vi "Untitled 6 (SubVI).vi"(0 "TestInterface in":refnum<class "TestInterface.lvclass">, 1 "timings":i32[](array[numeric]), 2 "reference 4":refnum<vi>, 3 "parameters":string[][](array[string]), 4 "reference 5":refnum<vi>, 5 "reference 6":refnum<vi>, 6 "reference 7":refnum<vi>, 8 "reference 3":refnum<vi>, 9 "name":string, 10 "response":bool[](array[boolean]), 11 "Command regex":string[](array[string]), 12 "reference 2":refnum<vi>, 13 "Commandlist":string, 14 "reference":refnum<vi>, 16 "wait":u32[](array[numeric])) -> (20 "TestInterface out":refnum<class "TestInterface.lvclass">, 27 "error out":errorcluster)   [LabVIEW 2013, in "DeviceInterface.lvclass"]
uses:
  DeviceInterface.lvclass
  Tests/TestInterface/TestInterface.lvclass
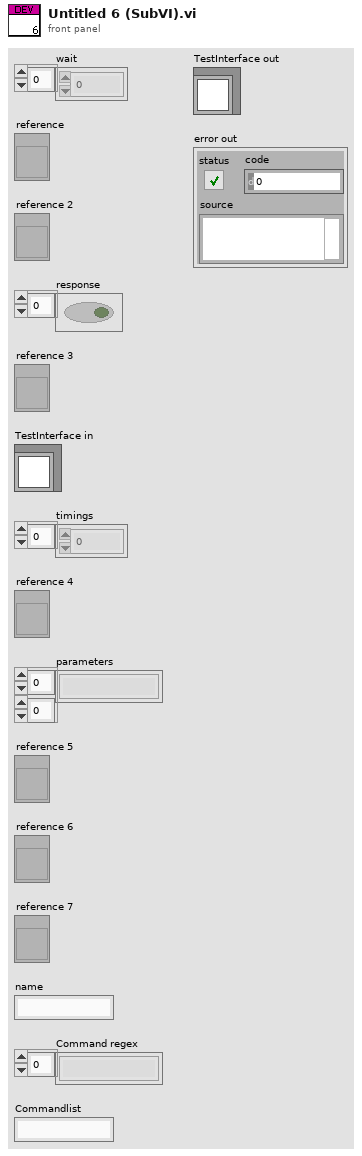
[diagram p1: front panel]
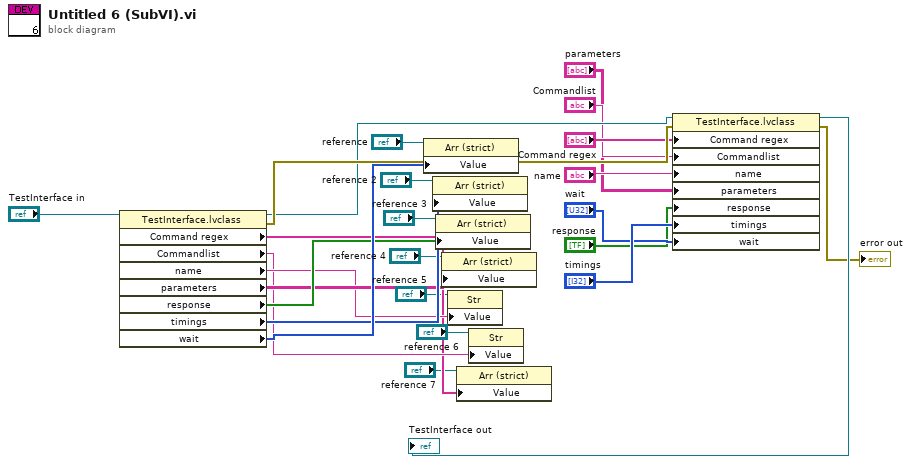
[diagram p0: block diagram]
diagram:
  n1 = property class="TestInterface.lvclass"(reference="TestInterface in") -> (reference out=w23:refnum<class "TestInterface.lvclass">, error out=w24:errorcluster, "Command regex"=w9:string[], "Commandlist"=w10:string, "name"=w11:string, "parameters"=w12:string[][], "response"=w13:bool[], "timings"=w14:i32[], "wait"=w15:u32[])  [unwired: 1 in]
  n2 = property class="Arr (strict)"(reference="reference", "Value"=w15) -> ()  [unwired: 1 in, 2 out]
  n3 = property class="Arr (strict)"(reference="reference 2", "Value"=w14) -> ()  [unwired: 1 in, 2 out]
  n4 = property class="Arr (strict)"(reference="reference 3", "Value"=w13) -> ()  [unwired: 1 in, 2 out]
  n5 = property class="Arr (strict)"(reference="reference 4", "Value"=w12) -> ()  [unwired: 1 in, 2 out]
  n6 = property class="Str"(reference="reference 5", "Value"=w11) -> ()  [unwired: 1 in, 2 out]
  n7 = property class="Arr (strict)"(reference="reference 7", "Value"=w9) -> ()  [unwired: 1 in, 2 out]
  n8 = property class="Str"(reference="reference 6", "Value"=w10) -> ()  [unwired: 1 in, 2 out]
  n9 = property class="TestInterface.lvclass"(reference=w23, error in=w24, "Command regex"="Command regex", "Commandlist"="Commandlist", "name"="name", "parameters"="parameters", "response"="response", "timings"="timings", "wait"="wait") -> (reference out=→"TestInterface out":refnum<class "TestInterface.lvclass">, error out=→"error out":errorcluster)
